vi "interpolate.vi"(10 "dy (mm)":dbl, 11 "initial array":dbl[][](array[numeric])) -> (2 "energy (eV)":dbl)   [LabVIEW 2014]
uses:
  <vilib>/gmath/NI_Gmath.lvlib
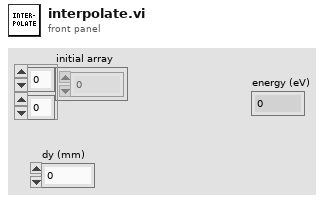
[diagram p1: front panel]
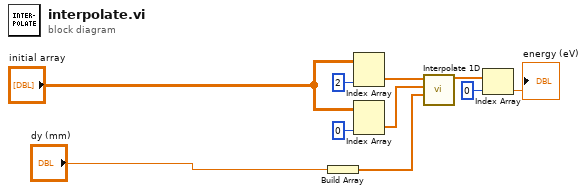
[diagram p0: block diagram]
diagram:
  n1 = Build Array("dy (mm)") -> (w4:dbl[])
  n2 = Index Array(array="initial array", index (col)=2 ("disabled index (col)")) -> (element=w8:dbl[])  [unwired: 1 in]
  n3 = Index Array(array="initial array", index (col)=0 ("disabled index (col)")) -> (element=w9:dbl[])  [unwired: 1 in]
  n4 = call <vilib>:"Interpolate 1D.vi"("xi"=w4, "X"=w9, "Y"=w8) -> ("yi"=w3:dbl[])  [unwired: 6 in, 2 out]
  n5 = Index Array(array=w3, index=0) -> (element=→"energy (eV)":dbl)
